vi "Do.vi"(8 "error in (no error)":errorcluster, 10 "Actor in":refnum<class "Actor.lvclass">, 11 "DNL_Message Template":refnum<class "Concrete Message Template.lvclass">) -> (0 "error out":errorcluster, 2 "Actor out":refnum<class "Actor.lvclass">)   [LabVIEW 2020, in "Concrete Message Template.lvclass"]
doc: "This VI delivers the message to the actor by calling the appropriate method(s) on the actor."
uses:
  Concrete Message Template.lvclass
  Concrete Message Template.lvclass/Concrete Message Template.ctl
  Abstract Message Template/Abstract Message Template.lvclass
  vi.lib/ActorFramework/Actor/Actor.lvclass
  34700b1e-4b1b-4205-ab4b-28631ba2a4c6.vi
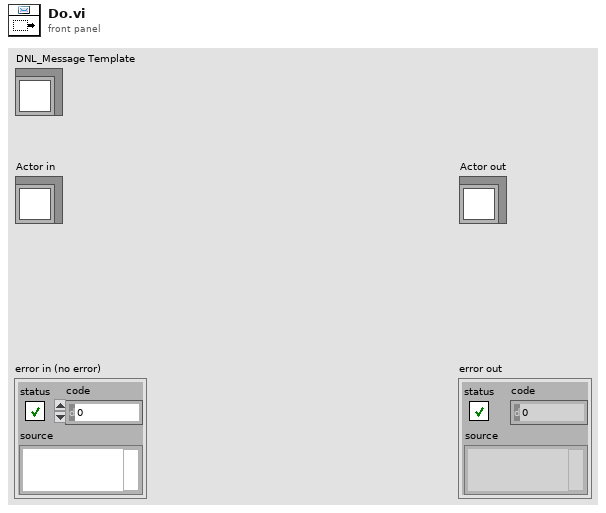
[diagram p1: front panel]
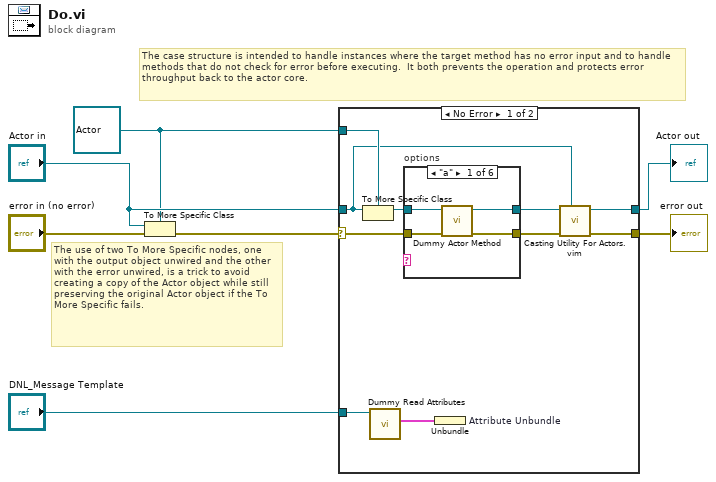
[diagram p0: block diagram]
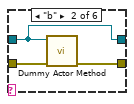
[diagram p2: hidden frame]
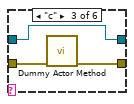
[diagram p3: hidden frame]
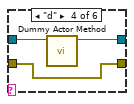
[diagram p4: hidden frame]
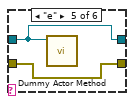
[diagram p5: hidden frame]
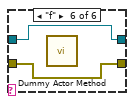
[diagram p6: hidden frame]
diagram:
  w2 = refnum<class "Actor.lvclass"> refnum ("Actor in")
  # "The use of two To More Specific nodes, one with the output object unwired and the other with the error unwired, is a trick to avoid creating a copy of the Actor object while still preserving the original Actor object if the To More Specific fails."
  # "The case structure is intended to handle instances where the target method has no error input and to handle methods that do not check for error before executing.  It both prevents the operation and protects error throughput back to the actor core."
  n1 = To More Specific Class(target class=w2, reference="Actor in", error in="error in (no error)") -> (error out=w6:errorcluster)  [unwired: 1 out]
  n2 = case shown="No Error" w6 {
    selector: w6 -> [w17 w36]
    tunnel: [w9 w36] -> w5
    tunnel: [w8 w35] -> w4
    tunnel: "Actor in" -> [w12 w35]
    tunnel: w2 -> [w13 _]
    tunnel: "DNL_Message Template" -> [w14 _]
    frame No Error {
      n3 = To More Specific Class(target class=w13, reference=w12) -> (specific class reference=w16:refnum<class "Actor.lvclass">)  [unwired: 1 in, 1 out]
      n4 = call "Dummy Read Attributes.vi"("Abstract Message Template in"=w14) -> ("Payload"=w15:cluster{})  [unwired: 9 in, 1 out]
      n5 = case "options" shown="\"a\"" {
        selector: _ -> [_ _ _ _ _ _]
        tunnel: [w21 w24 w27 w30 w31 w33] -> w10
        tunnel: [w20 w22 w25 w28 w32 w34] -> w11
        tunnel: w17 -> [w19 w23 w26 w30 w31 w33]
        tunnel: w16 -> [w18 w22 w25 w29 w32 w34]
        frame "a" {
          n6 = call "Dummy Actor Method.vi"("error in (no error)"=w19, "Actor in"=w18) -> ("error out"=w21:errorcluster, "Actor out"=w20:refnum<class "Actor.lvclass">)  [unwired: 8 in]
        }
        frame "b" {
          n7 = call "Dummy Actor Method.vi"("error in (no error)"=w23, "Actor in"=w22) -> ("error out"=w24:errorcluster)  [unwired: 8 in, 1 out]
        }
        frame "c" {
          n8 = call "Dummy Actor Method.vi"("error in (no error)"=w26) -> ("error out"=w27:errorcluster)  [unwired: 9 in, 1 out]
        }
        frame "d" {
          n9 = call "Dummy Actor Method.vi"("Actor in"=w29) -> ("Actor out"=w28:refnum<class "Actor.lvclass">)  [unwired: 9 in, 1 out]
        }
        frame "e" {
          n10 = call "Dummy Actor Method.vi"("Actor in"=w32) -> ()  [unwired: 9 in, 2 out]
        }
        frame "f" {
          n11 = call "Dummy Actor Method.vi"() -> ()  [unwired: 10 in, 2 out]
        }
      }
      n12 = Unbundle "Attribute Unbundle"(w15) -> ()  [unwired: 1 out]
      n13 = call "Casting Utility For Actors.vim"("type"=w12, "error in (no error)"=w10, "Actor in"=w11) -> ("error out"=w9:errorcluster, "Actor out"=w8:refnum<class "Actor.lvclass">)  [unwired: 7 in]
    }
    frame Error {
      # "If type check fails, pass the original object out again."
    }
  }
  "error out" <- w5
  "Actor out" <- w4
